vi "字符串.vi"() -> ()   [LabVIEW 2014]
panel:
  out "数字":dbl
  in  "数字字符串 2":string
  out "连接的字符串 2":string
  out "连接的字符串":string
  out "长度":i32
  in  "字符串":string
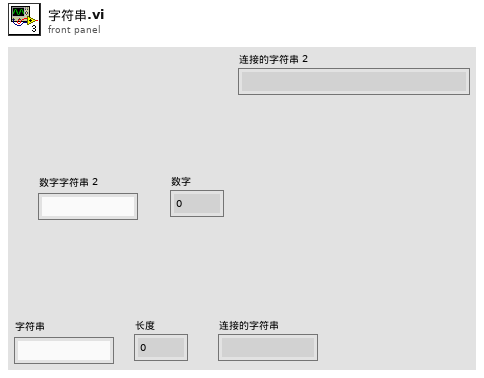
[diagram p1: front panel]
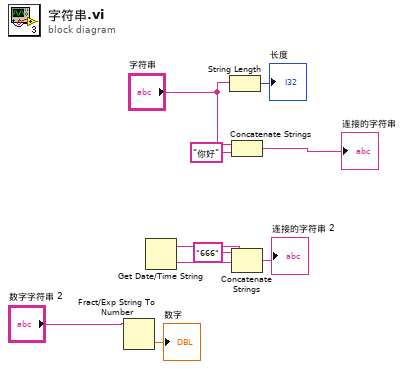
[diagram p0: block diagram]
diagram:
  n1 = Fract/Exp String To Number(string="数字字符串 2") -> (number=→"数字":dbl)  [unwired: 3 in, 1 out]
  n2 = Get Date/Time String() -> (date string=w6:string, time string=w5:string)  [unwired: 3 in]
  n3 = String Length(string="字符串") -> (length=→"长度":i32)
  n4 = Concatenate Strings("字符串", "你好" ("字符串")) -> (→"连接的字符串":string)
  n5 = Concatenate Strings(w6, w5, "666" ("字符串")) -> (→"连接的字符串 2":string)
